vi "setUp.vi"(8 "error in (no error)":errorcluster, 11 "reference in":refnum<class "DMA Channel Testing.lvclass">) -> (0 "error out":errorcluster, 3 "reference out":refnum<class "DMA Channel Testing.lvclass">)   [LabVIEW 2019, in "DMA Channel Testing.lvclass"]
doc: "setUp runs prior to the test method during test execution. Use this method to initialize any object data required by your tests."
uses:
  DMA Channel Testing.lvclass
  C:/Program Files (x86)/National Instruments/LabVIEW 2019/vi.lib/addons/_JKI Toolkits/VI Tester/TestCase.llb/TestCase.lvclass
  DMA Channel Testing.lvclass/DMA Channel Testing.ctl
  <vilib>/addons/_JKI Toolkits/VI Tester/TestCase.llb/TestCase.lvclass
  FPGA Addon Test Class/FPGA Addon Test Class.lvclass
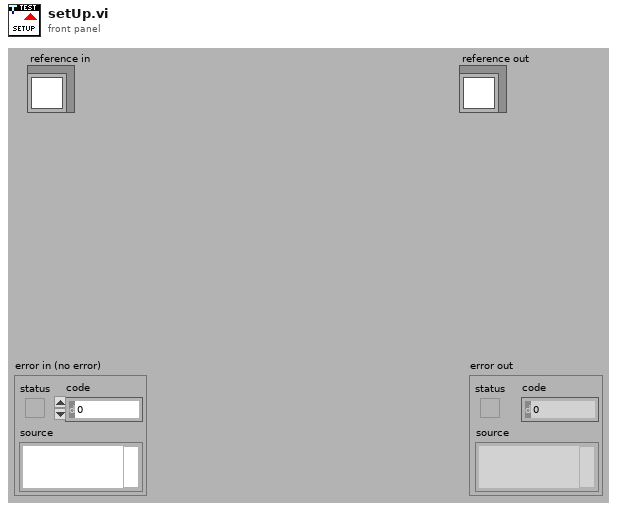
[diagram p1: front panel]
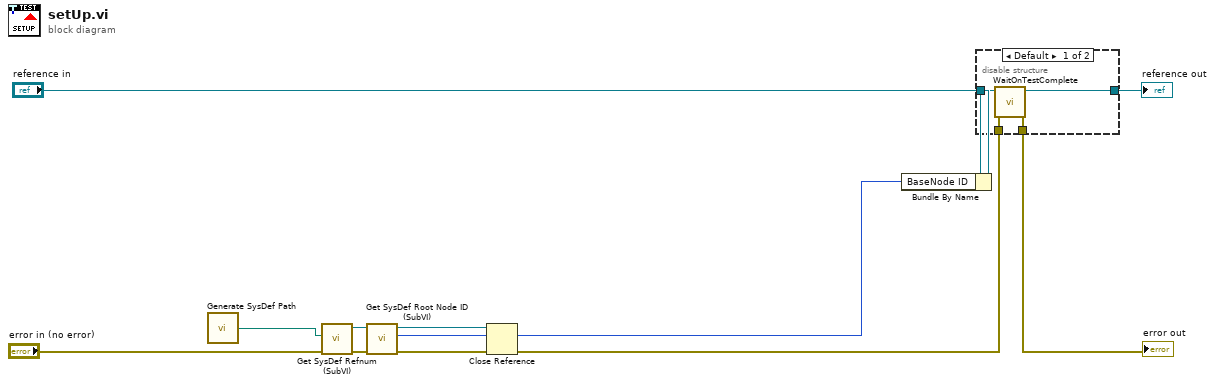
[diagram p0: block diagram]
diagram:
  n1 = call "Generate SysDef Path.vi"() -> ("System Definition path"=w1:path)
  n2 = call "Get SysDef Refnum (SubVI).vi"("error in (no error)"="error in (no error)", "System Definition path"=w1) -> ("error out"=w4:errorcluster, "SysDef Refnum out"=w3:refnum<k24>)  [unwired: 8 in]
  n3 = call "Get SysDef Root Node ID (SubVI).vi"("error in (no error)"=w4, "SysDef Refnum In"=w3) -> ("error out"=w7:errorcluster, "Root NodeID Out"=w8:u64, "SysDef Refnum Out"=w5:refnum<k24>)  [unwired: 7 in]
  n4 = Close Reference(reference=w5, error in (no error)=w7) -> (error out=w6:errorcluster)
  n5 = Bundle By Name(cluster="reference in", "BaseNode ID"=w8) -> (w9:refnum<class "DMA Channel Testing.lvclass">)
  n6 = disable-structure shown="Default" {
    disable-tunnel: w6 -> [w16 w17]
    disable-tunnel: [w15 w17] -> w12
    disable-tunnel: [w14 w18] -> w10
    disable-tunnel: w9 -> [w13 w18]
    frame condition #0 (active) {
      n7 = call <vilib>:"WaitOnTestComplete.vi"("error in (no error)"=w16, "TestCase in"=w13) -> ("error out"=w15:errorcluster, "TestCase out"=w14:refnum<class "DMA Channel Testing.lvclass">)  [unwired: 8 in]
    }
    frame condition #1 {
    }
  }
  "error out" <- w12
  "reference out" <- w10
